vi "GetMotorProperties.vi"(8 "error in (no error)":errorcluster, 9 "Channels":T1[](array[typedef]), 10 "Channel Properties":T2[](array[typedef])) -> (0 "error out":errorcluster, 2 "all exist":bool, 3 "Motor":T4)   [LabVIEW 2017, in "McsaAnalysisFunctions.lvlib"]
uses:
  <vilib>/addons/InsightCM/Utilities/Analysis/MCSA/McsaAnalysisFunctions.lvlib
  <vilib>/addons/InsightCM/Utilities/Analysis/MCSA/controls/McsaMotor.ctl
  <vilib>/addons/InsightCM/MessageBus/Base/controls/KeyValuePair.ctl
  <vilib>/addons/InsightCM/MessageBus/Base/controls/R2_Channel.ctl
  <vilib>/addons/InsightCM/MessageBus/Base/controls/Metric.ctl
  <vilib>/addons/InsightCM/Utilities/PropertyHelpers/PropertyHelpers.lvlib
  <vilib>/addons/InsightCM/Utilities/MCSA/McsaUtilities.lvlib
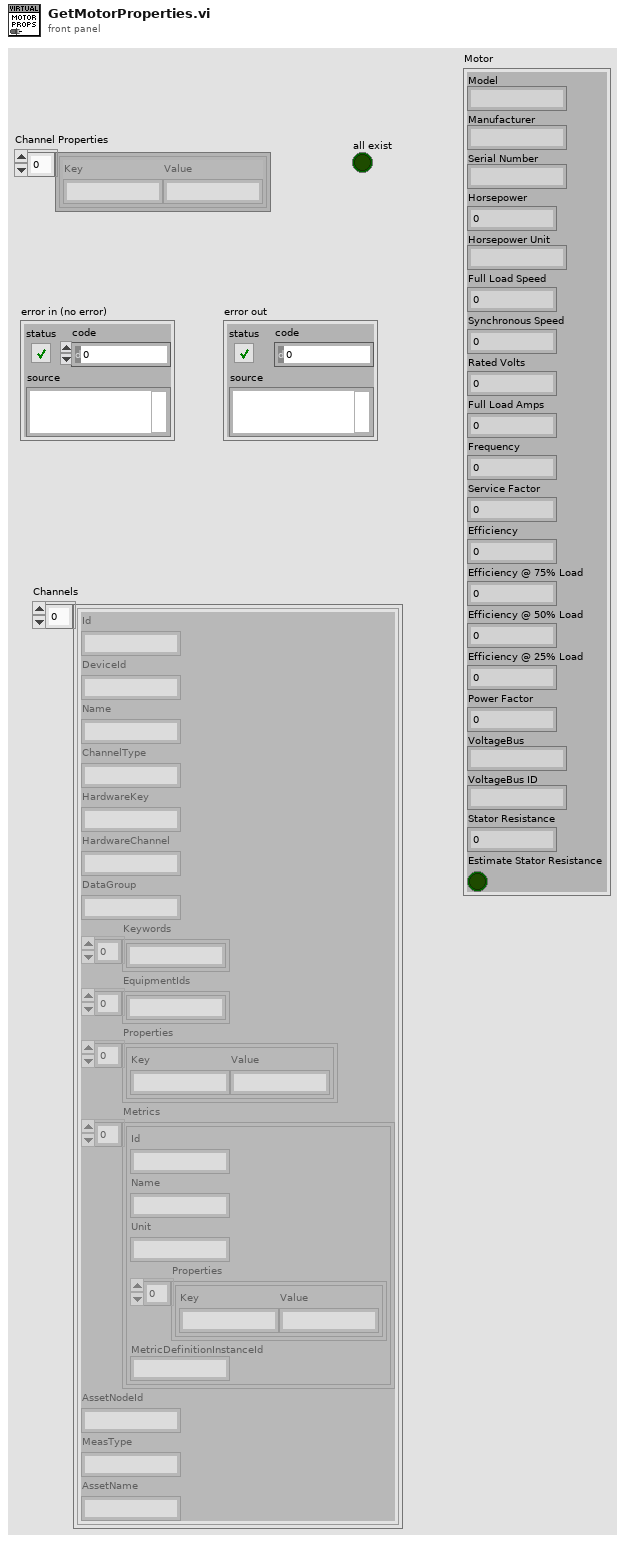
[diagram p1: front panel]
types:
  T1 = typedef "R2_Channel.ctl" = cluster{"Id":string, "DeviceId":string, "Name":string, "ChannelType":string, "HardwareKey":string, "HardwareChannel":string, "DataGroup":string, "Keywords":string[], "EquipmentIds":string[], "Properties":T2[], "Metrics":T3[], "AssetNodeId":string, "MeasType":string, "AssetName":string}
  T2 = typedef "KeyValuePair.ctl" = cluster{"Key":string, "Value":string}
  T3 = typedef "Metric.ctl" = cluster{"Id":string, "Name":string, "Unit":string, "Properties":T2[], "MetricDefinitionInstanceId":string}
  T4 = typedef "McsaAnalysisFunctions.lvlib/McsaMotor.ctl" = cluster{"Model":string, "Manufacturer":string, "Serial Number":string, "Horsepower":dbl, "Horsepower Unit":string, "Full Load Speed":dbl, "Synchronous Speed":dbl, "Rated Volts":dbl, "Full Load Amps":dbl, "Frequency":dbl, "Service Factor":dbl, "Efficiency":dbl, "Efficiency @ 75% Load":dbl, "Efficiency @ 50% Load":dbl, "Efficiency @ 25% Load":dbl, "Power Factor":dbl, "VoltageBus":string, "VoltageBus ID":string, "Stator Resistance":dbl, "Estimate Stator Resistance":bool}
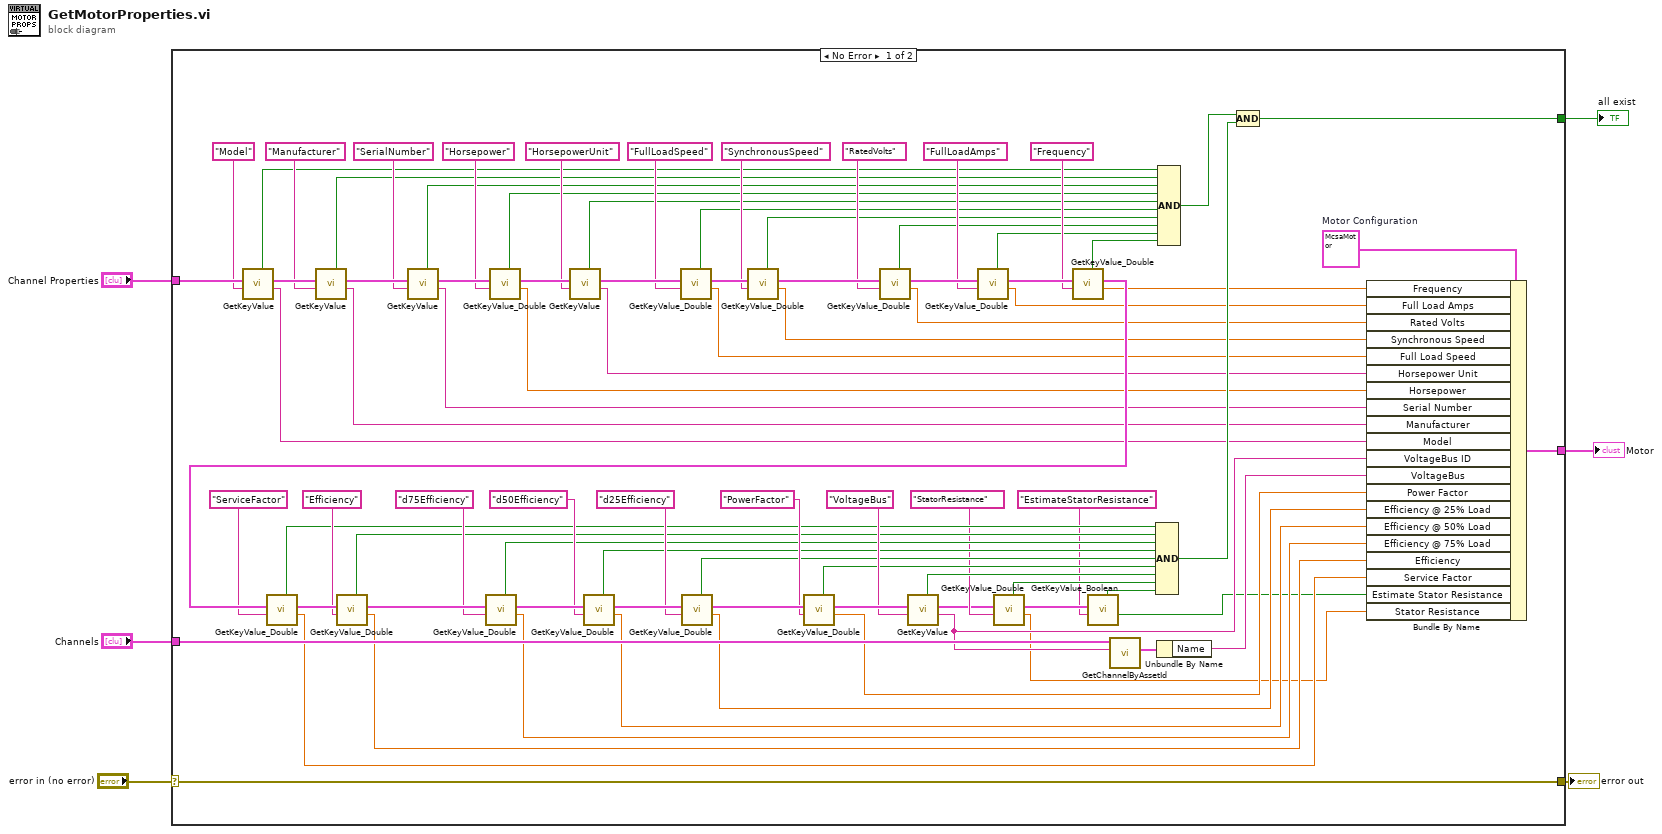
[diagram p0: block diagram]
diagram:
  n1 = case shown="No Error" "error in (no error)" {
    selector: "error in (no error)" -> [w16 w92]
    tunnel: "Channel Properties" -> [w91 _]
    tunnel: "Channels" -> [w56 _]
    tunnel: [w18 _] -> w4
    tunnel: [w17 _] -> w3
    tunnel: [w16 w92] -> w1
    frame No Error {
      w36 = T4 {"Model"="", "Manufacturer"="", "Serial Number"="", "Horsepower"=0.0, "Horsepower Unit"="", "Full Load Speed"=0.0, "Synchronous Speed"=0.0, "Rated Volts"=0.0, "Full Load Amps"=0.0, "Frequency"=0.0, "Service Factor"=0.0, "Efficiency"=0.0, "Efficiency @ 75% Load"=0.0, "Efficiency @ 50% Load"=0.0, "Efficiency @ 25% Load"=0.0, "Power Factor"=0.0, "VoltageBus"="", "VoltageBus ID"="", "Stator Resistance"=0.0, "Estimate Stator Resistance"=FALSE}  # Motor Configuration
      n2 = call <vilib>:"GetKeyValue.vi"("key"="Model" ("name"), "key value pairs"=w91) -> ("value"=w26:string, "key value pairs out"=w90:T2[], "found"=w55:bool)  [unwired: 7 in]
      n3 = call <vilib>:"GetKeyValue.vi"("key"="Manufacturer" ("name"), "key value pairs"=w90) -> ("value"=w27:string, "key value pairs out"=w89:T2[], "found"=w54:bool)  [unwired: 7 in]
      n4 = call <vilib>:"GetKeyValue.vi"("key"="SerialNumber" ("name"), "key value pairs"=w89) -> ("value"=w28:string, "key value pairs out"=w84:T2[], "found"=w53:bool)  [unwired: 7 in]
      n5 = call <vilib>:"GetKeyValue_Double.vi"("key"="Horsepower" ("name"), "key value pairs"=w84) -> ("value"=w29:dbl, "key value pairs out"=w85:T2[], "found"=w52:bool)  [unwired: 7 in]
      n6 = call <vilib>:"GetKeyValue.vi"("key"="HorsepowerUnit" ("name"), "key value pairs"=w85) -> ("value"=w30:string, "key value pairs out"=w81:T2[], "found"=w51:bool)  [unwired: 7 in]
      n7 = call <vilib>:"GetKeyValue_Double.vi"("key"="FullLoadSpeed" ("name"), "key value pairs"=w81) -> ("value"=w31:dbl, "key value pairs out"=w80:T2[], "found"=w50:bool)  [unwired: 7 in]
      n8 = call <vilib>:"GetKeyValue_Double.vi"("key"="SynchronousSpeed" ("name"), "key value pairs"=w80) -> ("value"=w32:dbl, "key value pairs out"=w79:T2[], "found"=w49:bool)  [unwired: 7 in]
      n9 = call <vilib>:"GetKeyValue_Double.vi"("key"="RatedVolts" ("name"), "key value pairs"=w79) -> ("value"=w33:dbl, "key value pairs out"=w78:T2[], "found"=w48:bool)  [unwired: 7 in]
      n10 = call <vilib>:"GetKeyValue_Double.vi"("key"="FullLoadAmps" ("name"), "key value pairs"=w78) -> ("value"=w34:dbl, "key value pairs out"=w77:T2[], "found"=w47:bool)  [unwired: 7 in]
      n11 = call <vilib>:"GetKeyValue_Double.vi"("key"="Frequency" ("name"), "key value pairs"=w77) -> ("value"=w35:dbl, "key value pairs out"=w70:T2[], "found"=w46:bool)  [unwired: 7 in]
      n12 = call <vilib>:"GetKeyValue_Double.vi"("key"="ServiceFactor" ("name"), "key value pairs"=w70) -> ("value"=w19:dbl, "key value pairs out"=w69:T2[], "found"=w44:bool)  [unwired: 7 in]
      n13 = call <vilib>:"GetKeyValue_Double.vi"("key"="Efficiency" ("name"), "key value pairs"=w69) -> ("value"=w20:dbl, "key value pairs out"=w68:T2[], "found"=w43:bool)  [unwired: 7 in]
      n14 = call <vilib>:"GetKeyValue_Double.vi"("key"="d75Efficiency" ("name"), "key value pairs"=w68) -> ("value"=w21:dbl, "key value pairs out"=w67:T2[], "found"=w42:bool)  [unwired: 7 in]
      n15 = call <vilib>:"GetKeyValue_Double.vi"("key"="d50Efficiency" ("name"), "key value pairs"=w67) -> ("value"=w22:dbl, "key value pairs out"=w66:T2[], "found"=w41:bool)  [unwired: 7 in]
      n16 = call <vilib>:"GetKeyValue_Double.vi"("key"="d25Efficiency" ("name"), "key value pairs"=w66) -> ("value"=w23:dbl, "key value pairs out"=w65:T2[], "found"=w40:bool)  [unwired: 7 in]
      n17 = call <vilib>:"GetKeyValue_Double.vi"("key"="PowerFactor" ("name"), "key value pairs"=w65) -> ("value"=w24:dbl, "key value pairs out"=w58:T2[], "found"=w39:bool)  [unwired: 7 in]
      n18 = call <vilib>:"GetKeyValue.vi"("key"="VoltageBus" ("name"), "key value pairs"=w58) -> ("value"=w15:string, "key value pairs out"=w13:T2[], "found"=w38:bool)  [unwired: 7 in]
      n19 = call <vilib>:"GetKeyValue_Double.vi"("key"="StatorResistance" ("name"), "key value pairs"=w13) -> ("value"=w11:dbl, "key value pairs out"=w10:T2[], "found"=w12:bool)  [unwired: 7 in]
      n20 = call <vilib>:"GetKeyValue_Boolean.vi"("key"="EstimateStatorResistance" ("name"), "key value pairs"=w10) -> ("value"=w8:bool, "found"=w7:bool)  [unwired: 7 in, 1 out]
      n21 = call <vilib>:"GetChannelByAssetId.vi"("node id"=w15, "channels in"=w56) -> ("channel"=w75:T1)  [unwired: 7 in, 2 out]
      n22 = Compound Arithmetic op=AND(w44, w43, w42, w41, w40, w39, w38, w12, w7) -> (w37:bool)
      n23 = Unbundle By Name(w75) -> ("Name"=w25:string)
      n24 = Compound Arithmetic op=AND(w55, w54, w53, w52, w51, w50, w49, w48, w47, w46) -> (w45:bool)
      n25 = Compound Arithmetic op=AND(w45, w37) -> (w17:bool)
      n26 = Bundle By Name(cluster=w36, "Frequency"=w35, "Full Load Amps"=w34, "Rated Volts"=w33, "Synchronous Speed"=w32, "Full Load Speed"=w31, "Horsepower Unit"=w30, "Horsepower"=w29, "Serial Number"=w28, "Manufacturer"=w27, "Model"=w26, "VoltageBus ID"=w15, "VoltageBus"=w25, "Power Factor"=w24, "Efficiency @ 25% Load"=w23, "Efficiency @ 50% Load"=w22, "Efficiency @ 75% Load"=w21, "Efficiency"=w20, "Service Factor"=w19, "Estimate Stator Resistance"=w8, "Stator Resistance"=w11) -> (w18:T4)
    }
    frame Error {
    }
  }
  "error out" <- w1
  "Motor" <- w4
  "all exist" <- w3
